vi "ma_SML One Shot Linear Weighting.vi"(0 "x(n)":dbl[](array[numeric]) format="%.2f", 1 "y(n-1)":dbl[](array[numeric]) format="%.2f", 2 "averaged sofar(n-1)":dbl, 3 "average size":dbl, 4 "reset?":bool) -> (5 "y(n)":dbl[](array[numeric]) format="%.2f", 6 "averaged sofar(n)":dbl)   [LabVIEW 2020, in "NI_MAPro.lvlib"]
uses:
  NI_MAPro.lvlib
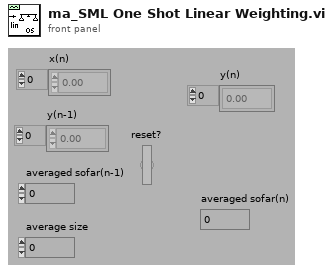
[diagram p1: front panel]
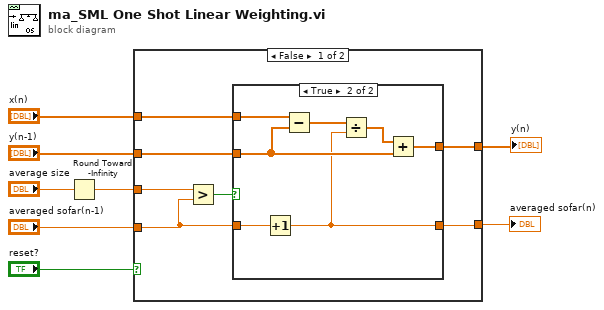
[diagram p0: block diagram]
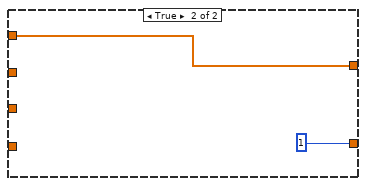
[diagram p3: hidden frame]
diagram:
  n1 = Round Toward -Infinity(1:"average size") -> (0:w1:dbl)
  n2 = case shown="False" "reset?" {
    tunnel: [w13 1] -> w7
    tunnel: [w10 w25] -> w5
    tunnel: "x(n)" -> [w12 w25]
    tunnel: "averaged sofar(n-1)" -> [w9 _]
    tunnel: w1 -> [w14 _]
    tunnel: "y(n-1)" -> [w11 _]
    frame False {
      n3 = Greater?(x=w14, y=w9) -> (0:w15:bool)
      n4 = case shown="True" w15 {
        tunnel: w9 -> [w16 w22]
        tunnel: [w16 w18] -> w13
        tunnel: w12 -> [_ w24]
        tunnel: w11 -> [w17 w20]
        tunnel: [w17 w19] -> w10
        frame False {
        }
        frame True {
          n5 = Increment(x=w22) -> (x+1=w18:dbl)
          n6 = Subtract(x=w24, y=w20) -> (x-y=w23:dbl[])
          n7 = Divide(x=w23, y=w18) -> (x/y=w21:dbl[])
          n8 = Add(x=w21, y=w20) -> (x+y=w19:dbl[])
        }
      }
    }
    frame True {
    }
  }
  "averaged sofar(n)" <- w7
  "y(n)" <- w5
